vi "libssh2_free.vi"(8 "error in (no error)":errorcluster, 10 "ptr":u64, 11 "session":T1) -> (0 "error out":errorcluster)   [LabVIEW 2013, in "libssh2.lvlib"]
doc: "Release memory allocated by earlier calls to libssh2 functions."
uses:
  libssh2.lvlib
  Session Refnum.ctl
  Global Settings.vi
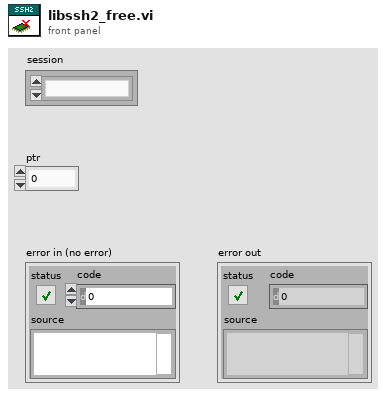
[diagram p1: front panel]
types:
  T1 = typedef "libssh2.lvlib/Session Refnum.ctl" = refnum<k1>
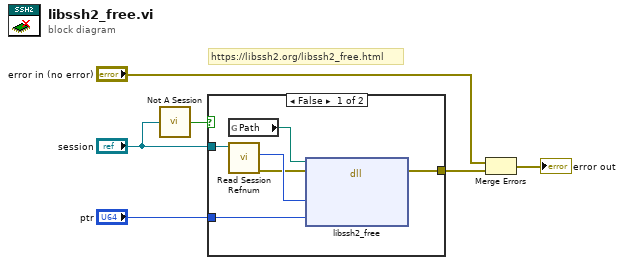
[diagram p0: block diagram]
diagram:
  # "https://libssh2.org/libssh2_free.html"
  n1 = call "Not A Session.vi"("session"="session") -> ("Not a Session?"=w3:bool)
  n2 = case shown="False" w3 {
    tunnel: [w11 _] -> w4
    tunnel: "session" -> [w10 _]
    tunnel: "ptr" -> [w7 _]
    frame False {
      n3 = global read "Global Settings.vi" "Path"() -> (w12:path)
      n4 = call "Read Session Refnum.vi"("session"=w10) -> ("error out"=w8:errorcluster, "LIBSSH2_SESSION*"=w9:u64)  [unwired: 6 in, 3 out]
      n5 = dll-call lib="?" fn="libssh2_free"(path in=w12, error in=w8, "session"=w9, "ptr"=w7) -> (error out=w11:errorcluster)  [unwired: 4 in, 1 out]
    }
    frame True {
    }
  }
  n6 = Merge Errors("error in (no error)", w4) -> (→"error out":errorcluster)
